vi "AI IRQ Preview.vi"(7 "Type":T1, 8 "error in (no error)":errorcluster, 9 "_Threhold Refnum":refnum<vi>, 10 "_Hysteresis Refnum":refnum<vi>, 11 "_Analog Preview Refnum":refnum<vi>) -> (0 "error out":errorcluster)   [LabVIEW 2021]
uses:
  <vilib>/myRIO/Common/Instrument Driver Framework/myRIO v1.0/IRQ/typedefs/AI IRQ Type.ctl
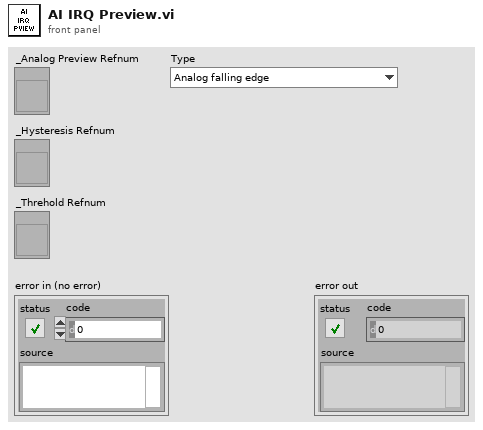
[diagram p1: front panel]
types:
  T1 = typedef "AI IRQ Type.ctl" = enum16{"Analog falling edge", "Analog rising edge"}
  T2 = typedef "LVCursorListTypeDef.ctl" = cluster{"Name":string, "Color":u32, "Style":u8, "Point Style":u8, "Name Visible":bool, "Allow Drag":bool, "Cursor Mode":u32, "Plot":i32, "Index":i32, "Position":cluster{"X":dbl, "Y":dbl}, "X Scale":u32, "Y Scale":u32, "Watch Plots":i32[], "Watch All Plots":bool, "Plot Area":i32, "Label Offset":cluster{"X":dbl, "Y":dbl}}[]
  T3 = cluster{"Name":string, "Color":u32, "Style":u8, "Point Style":u8, "Name Visible":bool, "Allow Drag":bool, "Cursor Mode":u32, "Plot":i32, "Index":i32, "Position":cluster{"X":dbl, "Y":dbl}, "X Scale":u32, "Y Scale":u32, "Watch Plots":i32[], "Watch All Plots":bool, "Plot Area":i32, "Label Offset":cluster{"X":dbl, "Y":dbl}}
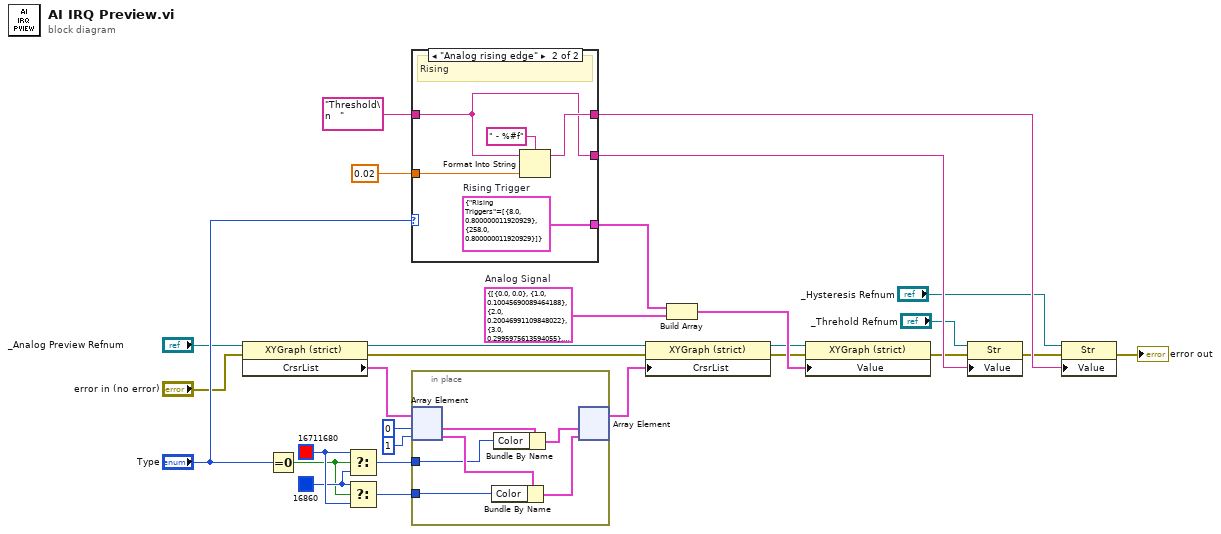
[diagram p0: block diagram]
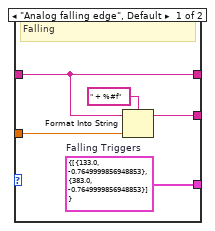
[diagram p2: hidden frame]
diagram:
  w1 = cluster{"Analog Signal":cluster{sgl, sgl}[]} {"Analog Signal"=[{0.0, 0.0}, {1.0, 0.1004569}, {2.0, 0.20046991}, {3.0, 0.29959756}, {4.0, 0.3974033}, {5.0, 0.4934578}, {6.0, 0.58734137}, {7.0, 0.67864627}, {8.0, 0.766979}, {9.0, 0.85196215}, {10.0, 0.933237}, {11.0, 1.010465}, {12.0, 1.08333}, {13.0, 1.1515396}, {14.0, 1.2148267}, {15.0, 1.2729516}, {16.0, 1.3257027}, {17.0, 1.3728974}, {18.0, 1.4143839}, {19.0, 1.4500413}, {20.0, 1.4797804}, {21.0, 1.5035442}, {22.0, 1.5213082}, {23.0, 1.5330803}, {24.0, 1.5389007}, {25.0, 1.5388417}, {26.0, 1.5330075}, {27.0, 1.5215328}, {28.0, 1.5045826}, {29.0, 1.4823511}, {30.0, 1.4550604}, {31.0, 1.422959}, {32.0, 1.386321}, {33.0, 1.3454434}, {34.0, 1.3006457}, {35.0, 1.2522669}, {36.0, 1.200664}, {37.0, 1.14621}, {38.0, 1.0892912}, {39.0, 1.0303059}, {40.0, 0.9696612}, {41.0, 0.907771}, {42.0, 0.8450537}, {43.0, 0.7819295}, {44.0, 0.71881837}, {45.0, 0.65613717}, {46.0, 0.5942976}, {47.0, 0.53370357}, {48.0, 0.4747491}, {49.0, 0.4178159}, {50.0, 0.36327127}, {51.0, 0.31146583}, {52.0, 0.26273167}, {53.0, 0.21738034}, {54.0, 0.17570114}, {55.0, 0.13795933}, {56.0, 0.10439472}, {57.0, 0.07522025}, {58.0, 0.050620776}, {59.0, 0.03075197}, {60.0, 0.015739478}, {61.0, 0.005678162}, {62.0, 0.0006315716}, {63.0, 0.0006315716}, {64.0, 0.005678162}, {65.0, 0.015739478}, {66.0, 0.03075197}, {67.0, 0.050620776}, {68.0, 0.07522025}, {69.0, 0.10439472}, {70.0, 0.13795933}, {71.0, 0.17570114}, {72.0, 0.21738034}, {73.0, 0.26273167}, {74.0, 0.31146583}, {75.0, 0.36327127}, {76.0, 0.4178159}, {77.0, 0.4747491}, {78.0, 0.53370357}, {79.0, 0.5942976}, {80.0, 0.65613717}, {81.0, 0.71881837}, {82.0, 0.7819295}, {83.0, 0.8450537}, {84.0, 0.907771}, {85.0, 0.9696612}, {86.0, 1.0303059}, {87.0, 1.0892912}, {88.0, 1.14621}, {89.0, 1.200664}, {90.0, 1.2522669}, {91.0, 1.3006457}, {92.0, 1.3454434}, {93.0, 1.386321}, {94.0, 1.422959}, {95.0, 1.4550604}, {96.0, 1.4823511}, {97.0, 1.5045826}, {98.0, 1.5215328}, {99.0, 1.5330075}, {100.0, 1.5388417}, {101.0, 1.5389007}, {102.0, 1.5330803}, {103.0, 1.5213082}, {104.0, 1.5035442}, {105.0, 1.4797804}, {106.0, 1.4500413}, {107.0, 1.4143839}, {108.0, 1.3728974}, {109.0, 1.3257027}, {110.0, 1.2729516}, {111.0, 1.2148267}, {112.0, 1.1515396}, {113.0, 1.08333}, {114.0, 1.010465}, {115.0, 0.933237}, {116.0, 0.85196215}, {117.0, 0.7669789}, {118.0, 0.67864627}, {119.0, 0.58734137}, {120.0, 0.4934578}, {121.0, 0.3974033}, {122.0, 0.29959756}, {123.0, 0.20046991}, {124.0, 0.1004569}, {125.0, -4.614788e-16}, {126.0, -0.1004569}, {127.0, -0.20046991}, {128.0, -0.29959756}, {129.0, -0.3974033}, {130.0, -0.4934578}, {131.0, -0.58734137}, {132.0, -0.67864627}, {133.0, -0.7669789}, {134.0, -0.85196215}, {135.0, -0.933237}, {136.0, -1.010465}, {137.0, -1.08333}, {138.0, -1.1515396}, {139.0, -1.2148267}, {140.0, -1.2729516}, {141.0, -1.3257027}, {142.0, -1.3728974}, {143.0, -1.4143839}, {144.0, -1.4500413}, {145.0, -1.4797804}, {146.0, -1.5035442}, {147.0, -1.5213082}, {148.0, -1.5330803}, {149.0, -1.5389007}, {150.0, -1.5388417}, {151.0, -1.5330075}, {152.0, -1.5215328}, {153.0, -1.5045826}, {154.0, -1.4823511}, {155.0, -1.4550604}, {156.0, -1.422959}, {157.0, -1.386321}, {158.0, -1.3454434}, {159.0, -1.3006457}, {160.0, -1.2522669}, {161.0, -1.200664}, {162.0, -1.14621}, {163.0, -1.0892912}, {164.0, -1.0303059}, {165.0, -0.9696612}, {166.0, -0.907771}, {167.0, -0.8450537}, {168.0, -0.7819295}, {169.0, -0.71881837}, {170.0, -0.65613717}, {171.0, -0.5942976}, {172.0, -0.53370357}, {173.0, -0.4747491}, {174.0, -0.4178159}, {175.0, -0.36327127}, {176.0, -0.31146583}, {177.0, -0.26273167}, {178.0, -0.21738034}, {179.0, -0.17570114}, {180.0, -0.13795933}, {181.0, -0.10439472}, {182.0, -0.07522025}, {183.0, -0.050620776}, {184.0, -0.03075197}, {185.0, -0.015739478}, {186.0, -0.005678162}, {187.0, -0.0006315716}, {188.0, -0.0006315716}, {189.0, -0.005678162}, {190.0, -0.015739478}, {191.0, -0.03075197}, {192.0, -0.050620776}, {193.0, -0.07522025}, {194.0, -0.10439472}, {195.0, -0.13795933}, {196.0, -0.17570114}, {197.0, -0.21738034}, {198.0, -0.26273167}, {199.0, -0.31146583}, {200.0, -0.36327127}, {201.0, -0.4178159}, {202.0, -0.4747491}, {203.0, -0.53370357}, {204.0, -0.5942976}, {205.0, -0.65613717}, {206.0, -0.71881837}, {207.0, -0.7819295}, {208.0, -0.8450537}, {209.0, -0.907771}, {210.0, -0.9696612}, {211.0, -1.0303059}, {212.0, -1.0892912}, {213.0, -1.14621}, {214.0, -1.200664}, {215.0, -1.2522669}, {216.0, -1.3006457}, {217.0, -1.3454434}, {218.0, -1.386321}, {219.0, -1.422959}, {220.0, -1.4550604}, {221.0, -1.4823511}, {222.0, -1.5045826}, {223.0, -1.5215328}, {224.0, -1.5330075}, {225.0, -1.5388417}, {226.0, -1.5389007}, {227.0, -1.5330803}, {228.0, -1.5213082}, {229.0, -1.5035442}, {230.0, -1.4797804}, {231.0, -1.4500413}, {232.0, -1.4143839}, {233.0, -1.3728974}, {234.0, -1.3257027}, {235.0, -1.2729516}, {236.0, -1.2148267}, {237.0, -1.1515396}, {238.0, -1.08333}, {239.0, -1.010465}, {240.0, -0.933237}, {241.0, -0.85196215}, {242.0, -0.7669789}, {243.0, -0.67864627}, {244.0, -0.58734137}, {245.0, -0.4934578}, {246.0, -0.3974033}, {247.0, -0.29959756}, {248.0, -0.20046991}, {249.0, -0.1004569}, {250.0, 1.4255446e-15}, {251.0, 0.1004569}, {252.0, 0.20046991}, {253.0, 0.29959756}, {254.0, 0.3974033}, {255.0, 0.4934578}, {256.0, 0.58734137}, {257.0, 0.67864627}, {258.0, 0.766979}, {259.0, 0.85196215}, {260.0, 0.933237}, {261.0, 1.010465}, {262.0, 1.08333}, {263.0, 1.1515396}, {264.0, 1.2148267}, {265.0, 1.2729516}, {266.0, 1.3257027}, {267.0, 1.3728974}, {268.0, 1.4143839}, {269.0, 1.4500413}, {270.0, 1.4797804}, {271.0, 1.5035442}, {272.0, 1.5213082}, {273.0, 1.5330803}, {274.0, 1.5389007}, {275.0, 1.5388417}, {276.0, 1.5330075}, {277.0, 1.5215328}, {278.0, 1.5045826}, {279.0, 1.4823511}, {280.0, 1.4550604}, {281.0, 1.422959}, {282.0, 1.386321}, {283.0, 1.3454434}, {284.0, 1.3006457}, {285.0, 1.2522669}, {286.0, 1.200664}, {287.0, 1.14621}, {288.0, 1.0892912}, {289.0, 1.0303059}, {290.0, 0.9696612}, {291.0, 0.907771}, {292.0, 0.8450537}, {293.0, 0.7819295}, {294.0, 0.71881837}, {295.0, 0.65613717}, {296.0, 0.5942976}, {297.0, 0.53370357}, {298.0, 0.4747491}, {299.0, 0.4178159}, {300.0, 0.36327127}, {301.0, 0.31146583}, {302.0, 0.26273167}, {303.0, 0.21738034}, {304.0, 0.17570114}, {305.0, 0.13795933}, {306.0, 0.10439472}, {307.0, 0.07522025}, {308.0, 0.050620776}, {309.0, 0.03075197}, {310.0, 0.015739478}, {311.0, 0.005678162}, {312.0, 0.0006315716}, {313.0, 0.0006315716}, {314.0, 0.005678162}, {315.0, 0.015739478}, {316.0, 0.03075197}, {317.0, 0.050620776}, {318.0, 0.07522025}, {319.0, 0.10439472}, {320.0, 0.13795933}, {321.0, 0.17570114}, {322.0, 0.21738034}, {323.0, 0.26273167}, {324.0, 0.31146583}, {325.0, 0.36327127}, {326.0, 0.4178159}, {327.0, 0.4747491}, {328.0, 0.53370357}, {329.0, 0.5942976}, {330.0, 0.65613717}, {331.0, 0.71881837}, {332.0, 0.7819295}, {333.0, 0.8450537}, {334.0, 0.907771}, {335.0, 0.9696612}, {336.0, 1.0303059}, {337.0, 1.0892912}, {338.0, 1.14621}, {339.0, 1.200664}, {340.0, 1.2522669}, {341.0, 1.3006457}, {342.0, 1.3454434}, {343.0, 1.386321}, {344.0, 1.422959}, {345.0, 1.4550604}, {346.0, 1.4823511}, {347.0, 1.5045826}, {348.0, 1.5215328}, {349.0, 1.5330075}, {350.0, 1.5388417}, {351.0, 1.5389007}, {352.0, 1.5330803}, {353.0, 1.5213082}, {354.0, 1.5035442}, {355.0, 1.4797804}, {356.0, 1.4500413}, {357.0, 1.4143839}, {358.0, 1.3728974}, {359.0, 1.3257027}, {360.0, 1.2729516}, {361.0, 1.2148267}, {362.0, 1.1515396}, {363.0, 1.08333}, {364.0, 1.010465}, {365.0, 0.933237}, {366.0, 0.85196215}, {367.0, 0.7669789}, {368.0, 0.67864627}, {369.0, 0.58734137}, {370.0, 0.4934578}, {371.0, 0.3974033}, {372.0, 0.29959756}, {373.0, 0.20046991}, {374.0, 0.1004569}, {375.0, -2.186065e-15}, {376.0, -0.1004569}, {377.0, -0.20046991}, {378.0, -0.29959756}, {379.0, -0.3974033}, {380.0, -0.4934578}, {381.0, -0.58734137}, {382.0, -0.67864627}, {383.0, -0.7669789}, {384.0, -0.85196215}, {385.0, -0.933237}, {386.0, -1.010465}, {387.0, -1.08333}, {388.0, -1.1515396}, {389.0, -1.2148267}, {390.0, -1.2729516}, {391.0, -1.3257027}, {392.0, -1.3728974}, {393.0, -1.4143839}, {394.0, -1.4500413}, {395.0, -1.4797804}, {396.0, -1.5035442}, {397.0, -1.5213082}, {398.0, -1.5330803}, {399.0, -1.5389007}, {400.0, -1.5388417}, {401.0, -1.5330075}, {402.0, -1.5215328}, {403.0, -1.5045826}, {404.0, -1.4823511}, {405.0, -1.4550604}, {406.0, -1.422959}, {407.0, -1.386321}, {408.0, -1.3454434}, {409.0, -1.3006457}, {410.0, -1.2522669}, {411.0, -1.200664}, {412.0, -1.14621}, {413.0, -1.0892912}, {414.0, -1.0303059}, {415.0, -0.9696612}, {416.0, -0.907771}, {417.0, -0.8450537}, {418.0, -0.7819295}, {419.0, -0.71881837}, {420.0, -0.65613717}, {421.0, -0.5942976}, {422.0, -0.53370357}, {423.0, -0.4747491}, {424.0, -0.4178159}, {425.0, -0.36327127}, {426.0, -0.31146583}, {427.0, -0.26273167}, {428.0, -0.21738034}, {429.0, -0.17570114}, {430.0, -0.13795933}, {431.0, -0.10439472}, {432.0, -0.07522025}, {433.0, -0.050620776}, {434.0, -0.03075197}, {435.0, -0.015739478}, {436.0, -0.005678162}, {437.0, -0.0006315716}, {438.0, -0.0006315716}, {439.0, -0.005678162}, {440.0, -0.015739478}, {441.0, -0.03075197}, {442.0, -0.050620776}, {443.0, -0.07522025}, {444.0, -0.10439472}, {445.0, -0.13795933}, {446.0, -0.17570114}, {447.0, -0.21738034}, {448.0, -0.26273167}, {449.0, -0.31146583}, {450.0, -0.36327127}, {451.0, -0.4178159}, {452.0, -0.4747491}, {453.0, -0.53370357}, {454.0, -0.5942976}, {455.0, -0.65613717}, {456.0, -0.71881837}, {457.0, -0.7819295}, {458.0, -0.8450537}, {459.0, -0.907771}, {460.0, -0.9696612}, {461.0, -1.0303059}, {462.0, -1.0892912}, {463.0, -1.14621}, {464.0, -1.200664}, {465.0, -1.2522669}, {466.0, -1.3006457}, {467.0, -1.3454434}, {468.0, -1.386321}, {469.0, -1.422959}, {470.0, -1.4550604}, {471.0, -1.4823511}, {472.0, -1.5045826}, {473.0, -1.5215328}, {474.0, -1.5330075}, {475.0, -1.5388417}, {476.0, -1.5389007}, {477.0, -1.5330803}, {478.0, -1.5213082}, {479.0, -1.5035442}, {480.0, -1.4797804}, {481.0, -1.4500413}, {482.0, -1.4143839}, {483.0, -1.3728974}, {484.0, -1.3257027}, {485.0, -1.2729516}, {486.0, -1.2148267}, {487.0, -1.1515396}, {488.0, -1.08333}, {489.0, -1.010465}, {490.0, -0.933237}, {491.0, -0.85196215}, {492.0, -0.7669789}, {493.0, -0.67864627}, {494.0, -0.58734137}, {495.0, -0.4934578}, {496.0, -0.3974033}, {497.0, -0.29959756}, {498.0, -0.20046991}, {499.0, -0.1004569}]}  # Analog Signal
  w19 = u32 16711680 ("Color")
  w18 = u32 16860 ("Color")
  n1 = property on="Property Node" class="XYGraph (strict)"(reference="_Analog Preview Refnum", error in="error in (no error)") -> (reference out=w8:refnum<vi>, error out=w24:errorcluster, "CrsrList"=w14:T2)
  n2 = Equal To 0?(x="Type") -> (x = 0?=w17:bool)
  n3 = Select(t=w19, s=w17, f=w18) -> (s? t:f=w20:u32)
  n4 = Select(t=w18, s=w17, f=w19) -> (s? t:f=w21:u32)
  n5 = case shown="\"Analog rising edge\"" "Type" {
    tunnel: [w29 w34] -> w25
    tunnel: "Threshold\n   " ("concatenated string") -> [w30 w35]
    tunnel: 0.02 ("input 1") -> [w33 w37]
    tunnel: [w31 w35] -> w28
    tunnel: [w30 w36] -> w27
    frame "Analog falling edge", Default {
      w29 = cluster{"Falling Triggers":cluster{sgl, sgl}[]} {"Falling Triggers"=[{133.0, -0.765}, {383.0, -0.765}]}  # Falling Triggers
      # "Falling"
      n6 = Format Into String(format string=" + %#f", initial string=w30, w33) -> (resulting string=w31:string)  [unwired: 1 in, 1 out]
    }
    frame "Analog rising edge" {
      w34 = cluster{"Rising Triggers":cluster{sgl, sgl}[]} {"Rising Triggers"=[{8.0, 0.8}, {258.0, 0.8}]}  # Rising Trigger
      # "Rising"
      n7 = Format Into String(format string=" - %#f", initial string=w35, w37) -> (resulting string=w36:string)  [unwired: 1 in, 1 out]
    }
  }
  n8 = in-place {
    in-place-border: w20 -> [w40]
    in-place-border: w21 -> [w39]
    n9 = in-place-array #1(w14, 0, 1) -> (w44:T3, w43:T3)
    n10 = Bundle By Name(cluster=w43, "Color"=w39) -> (w41:T3)
    n11 = Bundle By Name(cluster=w44, "Color"=w40) -> (w42:T3)
    n12 = in-place-array #1(w42, w41) -> (w15:T2)  [unwired: 2 out]
  }
  n13 = property on="Property Node" class="XYGraph (strict)"(reference=w8, error in=w24, "CrsrList"=w15) -> (reference out=w7:refnum<vi>, error out=w5:errorcluster)
  n14 = Build Array(w25, w1) -> (w26:cluster{"Analog Signal":cluster{sgl, sgl}[]}[])
  n15 = property on="Property Node" class="XYGraph (strict)"(reference=w7, error in=w5, "Value"=w26) -> (error out=w4:errorcluster)  [unwired: 1 out]
  n16 = property on="Property Node" class="Str"(reference="_Threhold Refnum", error in=w4, "Value"=w28) -> (error out=w3:errorcluster)  [unwired: 1 out]
  n17 = property on="Property Node" class="Str"(reference="_Hysteresis Refnum", error in=w3, "Value"=w27) -> (error out=→"error out":errorcluster)  [unwired: 1 out]
